vi "Configure Continuous Time Linear Equalizer Poles.vi"(7 "Pole Number (1: Pole 1)":u16(ring)=1 items=["Pole 1"=1, "Pole 2"=2, "Pole 3"=3], 8 "error in (no error)":errorcluster, 9 "Pole Frequency (1e+6 Hz)":dbl=1000000.0, 10 "Pole Count (0: Pole 2)":i32(ring) items=["Pole 2", "Pole 3"], 11 "VISA resource name":refnum<visa-resource-name>) -> (0 "error out":errorcluster, 3 "VISA resource name out":refnum<visa-resource-name>)   [LabVIEW 2020, in "Agilent 90000 Series.lvlib"]
doc: "Configures poles settings for continuous time linear equalizer."
uses:
  Agilent 90000 Series.lvlib
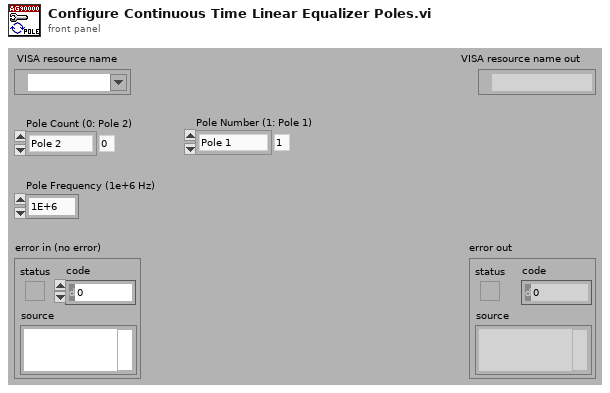
[diagram p1: front panel]
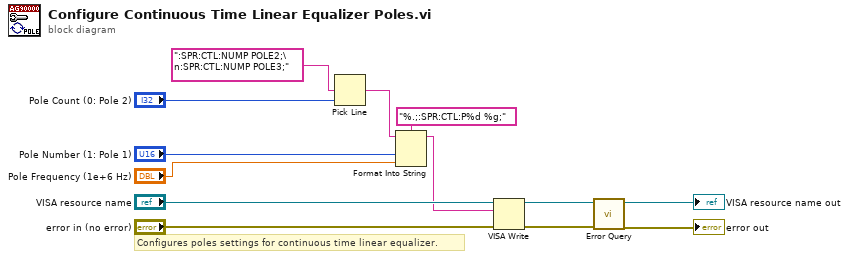
[diagram p0: block diagram]
diagram:
  # "Configures poles settings for continuous time linear equalizer."
  n1 = Pick Line(multi-line string=":SPR:CTL:NUMP POLE2;\n:SPR:CTL:NUMP POLE3;", line index="Pole Count (0: Pole 2)") -> (output string=w5:string)  [unwired: 1 out]
  n2 = Format Into String(format string="%.;:SPR:CTL:P%d %g;", initial string=w5, "Pole Number (1: Pole 1)", "Pole Frequency (1e+6 Hz)") -> (resulting string=w4:string)  [unwired: 1 in, 1 out]
  n3 = VISA Write(VISA resource name="VISA resource name", write buffer=w4, error in (no error)="error in (no error)") -> (VISA resource name out=w9:refnum<visa-resource-name>, error out=w8:errorcluster)  [unwired: 1 out]
  n4 = call "Error Query.vi"("error in (no error)"=w8, "VISA resource name"=w9) -> ("error out"=→"error out":errorcluster, "VISA resource name out"=→"VISA resource name out":refnum<visa-resource-name>)  [unwired: 8 out]
